vi "Wait.vi"(7 "Result Type (Variant)":refnum<class>, 8 "error in (no error)":errorcluster, 9 "Timeout mS (-1)":i32=-1, 11 "Future in":refnum<class "Future.lvclass">) -> (0 "error out":errorcluster, 2 "Result":refnum<class>)   [LabVIEW 2020, in "Promises.lvlib" / "Future.lvclass"]
doc: "Waits for the Future, and any Promise chaining if applied to the Future, to be resolved with a value from the task writing to the Promise. If chaining has been applied to the Future, this VI will also propagate results between tasks until the last task in the chain completes.\n\nIf a task resolves the Promise with an error, that error will be returned here. A value can only be read from a Future once. As soon as the value is read from the Future, the Future becomes invalid.\n\nIf progress should be made on the Promise chain without blocking, <b>Try Step.vi</b> can be used instead."
uses:
  Future.lvclass
  Future.lvclass/Future.ctl
  Promise/Promise.lvclass/Promise.ctl
  0a4c69f8-5422-426c-9c43-7ea82bc8a8e8.vi
  Create.vi
  Variant/Variant.lvclass
  Promise/Promise.lvclass
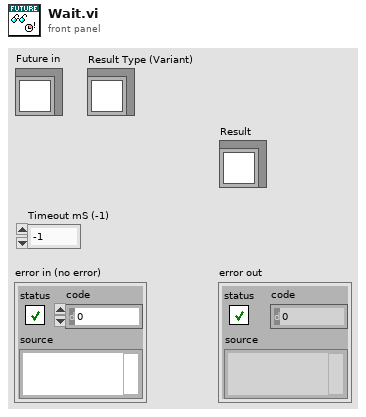
[diagram p1: front panel]
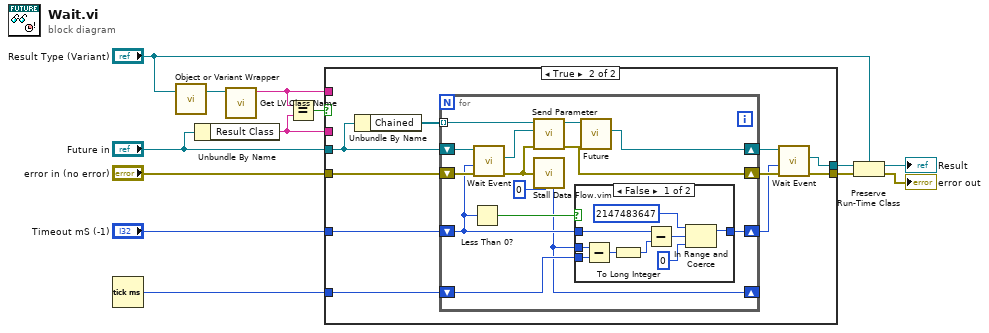
[diagram p0: block diagram]
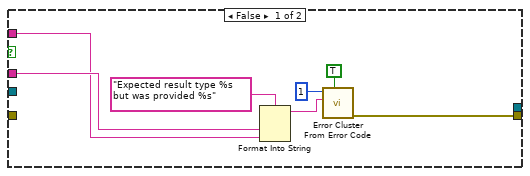
[diagram p2: hidden frame]
diagram:
  n1 = Tick Count (ms)() -> (millisecond timer value=w2:u32)
  n2 = call "Object or Variant Wrapper.vi"("LabVIEW Object"="Result Type (Variant)") -> ("Object or Variant Wrapper"=w1:refnum<class>)  [unwired: 6 in]
  n3 = Unbundle By Name("Future in") -> ("Result Class"=w4:string)
  n4 = call <vilib>:"Get LV Class Name.vi"("object"=w1) -> ("class name"=w5:string)  [unwired: 9 in, 1 out]
  n5 = Equal?(x=w5, y=w4) -> (x = y?=w11:bool)
  n6 = case shown="True" w11 {
    tunnel: "Future in" -> [_ w28]
    tunnel: "Timeout mS (-1)" -> [_ w29]
    tunnel: "error in (no error)" -> [_ w30]
    tunnel: [_ w22] -> w8
    tunnel: [w20 w23] -> w7
    tunnel: w5 -> [w15 _]
    tunnel: w4 -> [w16 _]
    tunnel: w2 -> [_ w25]
    frame False {
      n7 = Format Into String(format string="Expected result type %s but was provided %s", w16, w15) -> (resulting string=w14:string)  [unwired: 2 in, 1 out]
      n8 = call <vilib>:"Error Cluster From Error Code.vi"("show call chain? (False)"=TRUE, "error message (\"\")"=w14, "error code (0)"=1) -> ("error out"=w20:errorcluster)  [unwired: 6 in]
    }
    frame True {
      n9 = Unbundle By Name(w28) -> ("Chained"=w21:refnum<class "Promise.lvclass">[])
      n10 = for {
        shift-right: [w39] -> w27
        shift-left: w28 -> [w43]
        tunnel: w21 -> [w42] mode=indexing
        shift-right: [w32] -> w26
        shift-left: w30 -> [w44]
        shift-right: [w36] -> w24
        shift-left: w29 -> [w35]
        shift-right: [w31] -> _
        shift-left: w25 -> [w38]
        n11 = Less Than 0?(x=w35) -> (x < 0?=w34:bool)
        n12 = call "Wait Event.vi"("error in (no error)"=w44, "Timeout mS (-1)"=w35, "Future in"=w43) -> ("error out"=w33:errorcluster, "Value"=w41:refnum<class>)  [unwired: 5 in, 2 out]
        n13 = call "Send Parameter.vi"("error in (no error)"=w33, "Parameter"=w41, "Promise in"=w42) -> ("error out"=w32:errorcluster, "Promise out"=w40:refnum<class "Promise.lvclass">)  [unwired: 7 in]
        n14 = call "Stall Data Flow.vim"("value in"=w33, "milliseconds to wait"=u32 0) -> ("millisecond timer value"=w31:u32)  [unwired: 1 out]
        n15 = case shown="False" w34 {
          tunnel: w38 -> [w53 _]
          tunnel: w31 -> [w52 _]
          tunnel: [w46 w54] -> w36
          tunnel: w35 -> [w49 w54]
          frame False {
            n16 = Subtract(x=w52, y=w53) -> (x-y=w51:u32)
            n17 = To Long Integer(number=w51) -> (32bit integer=w50:i32)
            n18 = Subtract(x=w49, y=w50) -> (x-y=w48:i32)
            n19 = In Range and Coerce(upper limit=2147483647, x=w48, lower limit=0) -> (coerced(x)=w46:i32)  [unwired: 1 out]
          }
          frame True {
          }
        }
        n20 = call "Future.vi"("Promise in"=w40) -> ("Future"=w39:refnum<class "Future.lvclass">)  [unwired: 9 in, 1 out]
      }
      n21 = call "Wait Event.vi"("error in (no error)"=w26, "Timeout mS (-1)"=w24, "Future in"=w27) -> ("error out"=w23:errorcluster, "Value"=w22:refnum<class>)  [unwired: 5 in, 2 out]
    }
  }
  n22 = Preserve Run-Time Class(object in=w8, error in=w7, 2:"Result Type (Variant)") -> (object out=→"Result":refnum<class>, error out=→"error out":errorcluster)
